vi "AlliGator Get Pile-up Correction Parameter.vi"(8 "error in (no error)":errorcluster, 9 "Pixel Well Capacity in":u32, 10 "Pile-up Correction in":bool, 11 "Data Information":string) -> (0 "error out":errorcluster, 1 "Pixel Well Capacity out":u32, 2 "Pile-up Correction out":bool, 3 "Pile-up Correction (already) applied?":bool)   [LabVIEW 2021, in "AlliGator HDF5.lvlib"]
doc: "Reads from the metadata whether or not pile-up correction was already applied, and if so, does not repeat it."
uses:
  AlliGator HDF5.lvlib
panel:
  # "see the AlliGator License on the block diagram (Ctrl+E or Window:Show Block Diagram)"
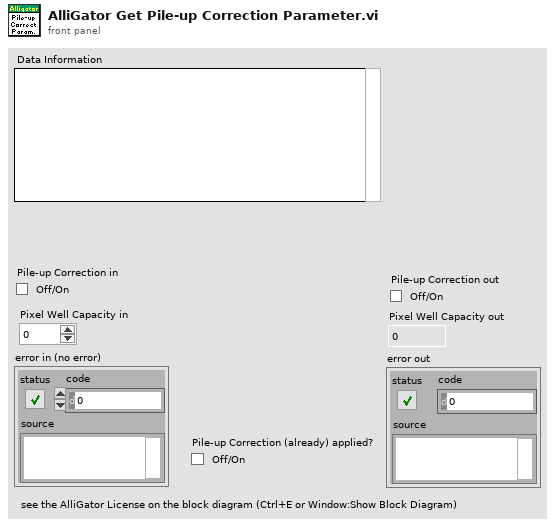
[diagram p1: front panel]
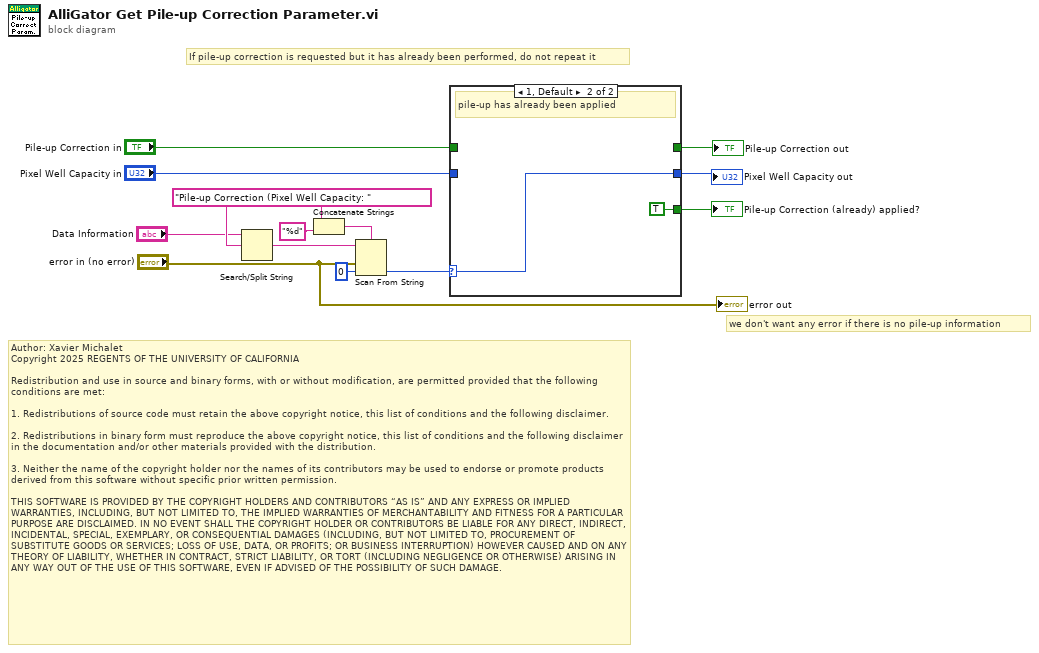
[diagram p0: block diagram]
diagram:
  w11 = "Pile-up Correction (Pixel Well Capacity: " ("format string")
  # "Author: Xavier Michalet\nCopyright 2025 REGENTS OF THE UNIVERSITY OF CALIFORNIA\n\nRedistribution and use in source and binary forms, with or without modification, are permitted provided that the following conditions are met:\n\n1. Redistributions of source code must retain the above copyright notice, this list of conditions and the following disclaimer.\n\n2. Redistributions in binary form must reproduce the above copyright notice, this list of conditions and the following disclaimer in the documentation and/or other materials provided with the distribution.\n\n3. Neither the name of the copyright holder nor the names of its contributors may be used to endorse or promote products derived from this software without specific prior written permission.\n\nTHIS SOFTWARE IS PROVIDED BY THE COPYRIGHT HOLDERS AND CONTRIBUTORS “AS IS” AND ANY EXPRESS OR IMPLIED WARRANTIES, INCLUDING, BUT NOT LIMITED TO, THE IMPLIED WARRANTIES OF MERCHANTABILITY AND FITNESS FOR A PARTICULAR PURPOSE ARE DISCLAIMED. IN NO EVENT SHALL THE COPYRIGHT HOLDER OR CONTRIBUTORS BE LIABLE FOR ANY DIRECT, INDIRECT, INCIDENTAL, SPECIAL, EXEMPLARY, OR CONSEQUENTIAL DAMAGES (INCLUDING, BUT NOT LIMITED TO, PROCUREMENT OF SUBSTITUTE GOODS OR SERVICES; LOSS OF USE, DATA, OR PROFITS; OR BUSINESS INTERRUPTION) HOWEVER CAUSED AND ON ANY THEORY OF LIABILITY, WHETHER IN CONTRACT, STRICT LIABILITY, OR TORT (INCLUDING NEGLIGENCE OR OTHERWISE) ARISING IN ANY WAY OUT OF THE USE OF THIS SOFTWARE, EVEN IF ADVISED OF THE POSSIBILITY OF SUCH DAMAGE."
  # "If pile-up correction is requested but it has already been performed, do not repeat it"
  # "we don't want any error if there is no pile-up information"
  n1 = Search/Split String(string="Data Information", search string/char (-)=w11) -> (match + rest of string=w9:string)  [unwired: 1 in, 2 out]
  n2 = Concatenate Strings(w11, "%d" ("string")) -> (w13:string)
  n3 = Scan From String(format string=w13, input string=w9, error in="error in (no error)", default 1=u32 0 ("default value 1")) -> (output 1=w6:u32)  [unwired: 1 in, 3 out]
  n4 = case shown="1, Default" w6 {
    selector: w6 -> [_ w17]
    tunnel: "Pile-up Correction in" -> [w14 _]
    tunnel: [w14 _] -> w4
    tunnel: "Pixel Well Capacity in" -> [w15 _]
    tunnel: [w15 w17] -> w2
    tunnel: [w14 TRUE ("Pile-up Correction in")] -> w1
    frame 0 {
      # "pile-up was not applied"
    }
    frame 1, Default {
      # "pile-up has already been applied"
    }
  }
  "Pixel Well Capacity out" <- w2
  "Pile-up Correction out" <- w4
  "Pile-up Correction (already) applied?" <- w1
  "error out" <- "error in (no error)"
